vi "Number Loop.vi"(2 "Step":i64, 7 "In":i64) -> (8 "Out":i64)   [LabVIEW 2010]
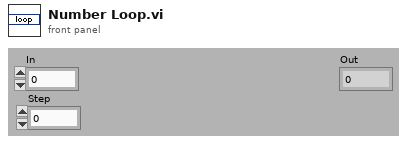
[diagram p1: front panel]
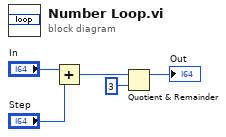
[diagram p0: block diagram]
diagram:
  n1 = Add(x="In", y="Step") -> (x+y=w2:i64)
  n2 = Quotient & Remainder(x=w2, y=3) -> (x-y*floor(x/y)=→"Out":i64)  [unwired: 1 out]
